vi "Sys config window-Set disabled states.vi"(8 "error in (no error)":errorcluster) -> (0 "error out":errorcluster)   [LabVIEW 2020]
uses:
  Globals/Sys Config window globals.vi
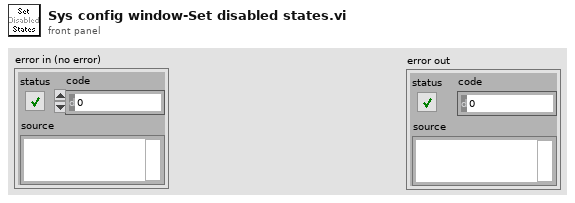
[diagram p1: front panel]
types:
  T1 = enum8{"Enabled", "Disabled", "Disabled and Grayed Out"}
  T2 = typedef "HW config window refs cluster.ctl" = cluster{"VI's reference":refnum<vi>, "menu reference":refnum<k9>, "Pane":refnum<vi>, "Config Tab Control":refnum<vi>, "Triggers sub-tab control":refnum<vi>, "Microscope ID":refnum<vi>, "Microscope Type":refnum<vi>, "Revision Number":refnum<vi>, "Advanced Imaging":refnum<vi>, "Max Allowed Trial Length":refnum<vi>, "Initial Scan Resolution":refnum<vi>, "Initial Acceptance Angle":refnum<vi>, "Initial Laser Wavelength [nm] ":refnum<vi>, "Initial Dwell Time [us]":refnum<vi>, "Error Logging":refnum<vi>, "Performance Monitoring":refnum<vi>, "Ctrl FPGA available":refnum<vi>, "Control HW config":refnum<vi>, "Control System Config":refnum<vi>, "General trigger settings":refnum<vi>, "Trigger HW config":refnum<vi>, "Externalise Triggers":refnum<vi>, "[Triggers output setup]":refnum<vi>, "DAQ FPGA HW Config":refnum<vi>, "DAQ FPGA System Config":refnum<vi>, "Pockels AO":refnum<vi>, "Hard shutter AO":refnum<vi>, "PMT AOs":refnum<vi>, "Galvo AO":refnum<vi>, "Power meter AI":refnum<vi>, "PMT Voltage Lower Limit":refnum<vi>, "PMT Voltage Upper Limit":refnum<vi>, "XYZ Stage Control Config":refnum<vi>, "XY stage available":refnum<vi>, "XY Comms Config Cluster":refnum<vi>, "Y stage available":refnum<vi>, "Y Comms Config Cluster":refnum<vi>, "Z stage available":refnum<vi>, "Z Comms Config Cluster":refnum<vi>, "Encoder available":refnum<vi>, "Encoder":refnum<vi>, "Encoder IP address":refnum<vi>, "Encoder port":refnum<vi>, "Wheel radius (cm)":refnum<vi>, "Demo mode":refnum<vi>, "Swap XY on stage":refnum<vi>, "Number of AODs":refnum<vi>, "Axial MC Supported":refnum<vi>, "MC Supported":refnum<vi>, "Computer MAC add.":refnum<vi>, "Cam VidRec available":refnum<vi>, "Cam VidRec":refnum<vi>, "DO flag-Video record":refnum<vi>, "DO flag-Trial start":refnum<vi>, "AOD Settings (distilled)":refnum<vi>, "Pockels cal.Dwell time (µs)":refnum<vi>, "Pockels cal.Zoom":refnum<vi>, "Current Objective":refnum<vi>, "[Obj. Calib. Settings]":refnum<vi>, "Laser Wavelength":refnum<vi>, "Laser Power Control \nHW config":refnum<vi>, "Laser 1 available":refnum<vi>, "Laser 1 config":refnum<vi>, "Prechirper 1 available":refnum<vi>, "Prechirper 1 config":refnum<vi>, "PreChirp Preset Values":refnum<vi>, "[PreChirper Preset \nCalibration Values]":refnum<vi>, "Prechirper Constants":refnum<vi>}
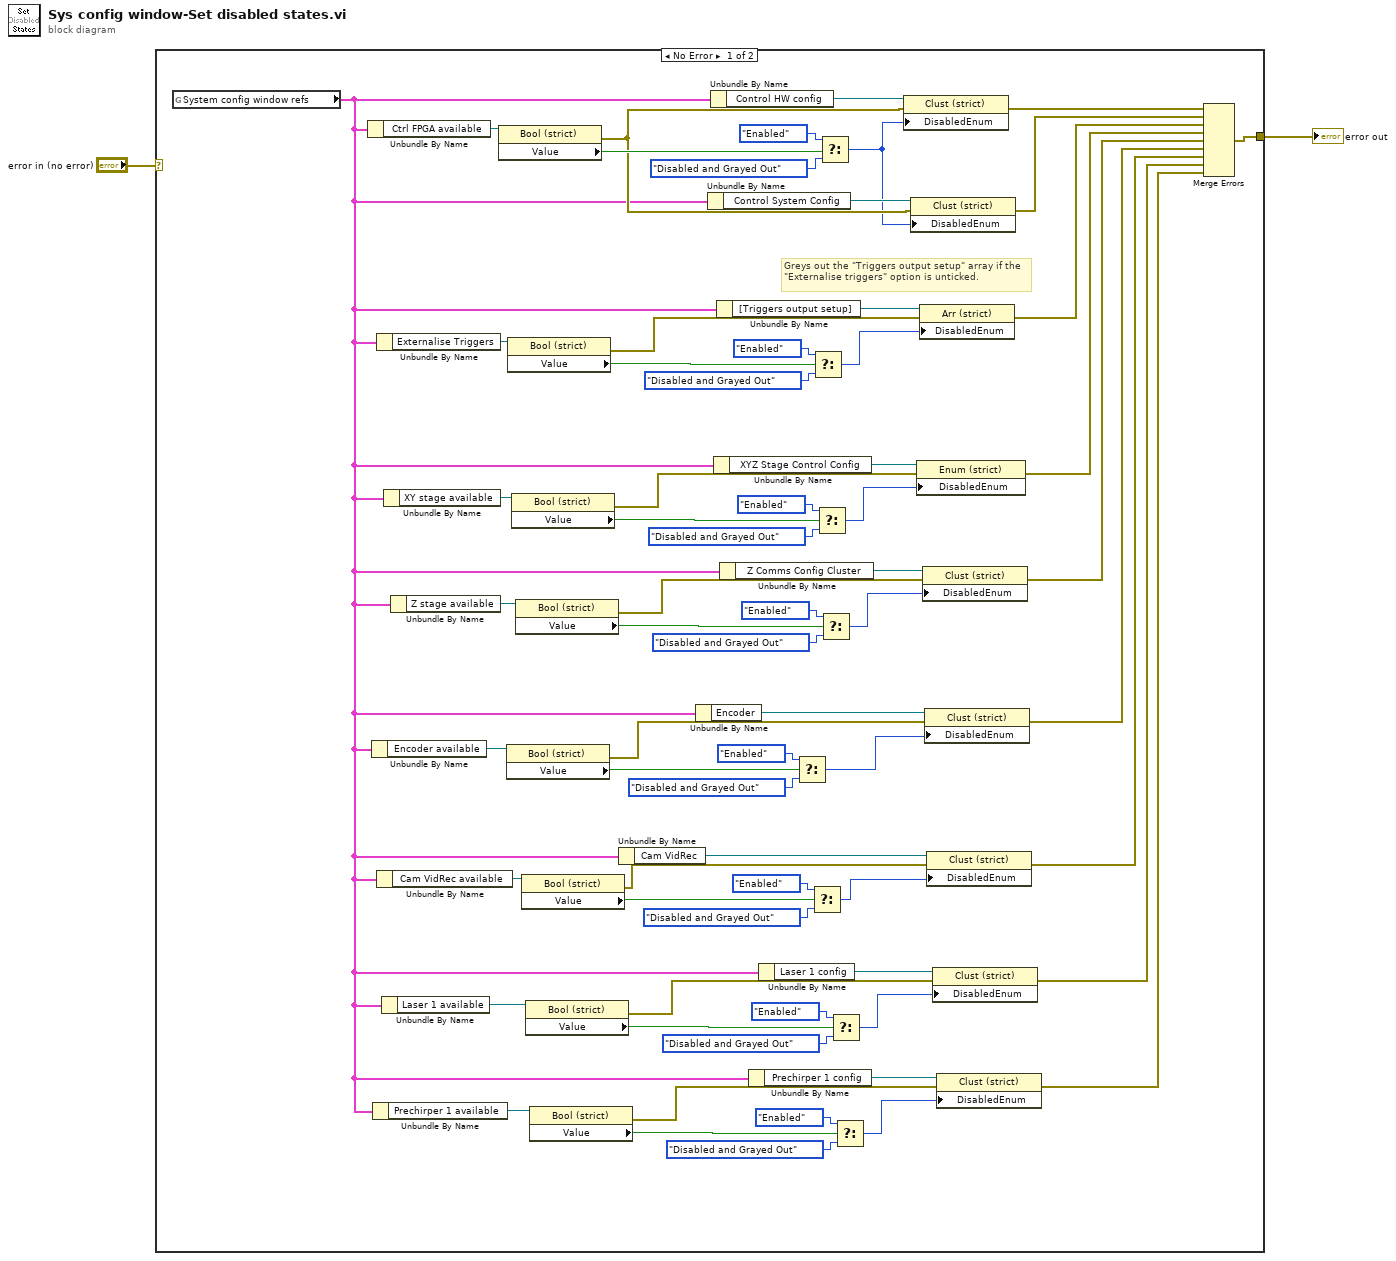
[diagram p0: block diagram]
diagram:
  n1 = case shown="No Error" "error in (no error)" {
    selector: "error in (no error)" -> [_ w71]
    tunnel: [w58 w71] -> w2
    frame No Error {
      # "Greys out the \"Triggers output setup\" array if the \"Externalise triggers\" option is unticked."
      n2 = global read "Sys Config window globals.vi" "System config window refs"() -> (w5:T2)
      n3 = Unbundle By Name(w5) -> ("Ctrl FPGA available"=w47:refnum<vi>)
      n4 = Unbundle By Name(w5) -> ("Encoder available"=w57:refnum<vi>)
      n5 = Unbundle By Name(w5) -> ("Prechirper 1 available"=w23:refnum<vi>)
      n6 = Unbundle By Name(w5) -> ("Externalise Triggers"=w70:refnum<vi>)
      n7 = Unbundle By Name(w5) -> ("Cam VidRec available"=w60:refnum<vi>)
      n8 = Unbundle By Name(w5) -> ("Laser 1 available"=w22:refnum<vi>)
      n9 = Unbundle By Name(w5) -> ("XY stage available"=w39:refnum<vi>)
      n10 = Unbundle By Name(w5) -> ("Z stage available"=w38:refnum<vi>)
      n11 = property class="Bool (strict)"(reference=w47) -> (error out=w6:errorcluster, "Value"=w46:bool)  [unwired: 1 in, 1 out]
      n12 = property class="Bool (strict)"(reference=w57) -> (error out=w51:errorcluster, "Value"=w56:bool)  [unwired: 1 in, 1 out]
      n13 = property class="Bool (strict)"(reference=w70) -> (error out=w64:errorcluster, "Value"=w68:bool)  [unwired: 1 in, 1 out]
      n14 = property class="Bool (strict)"(reference=w39) -> (error out=w45:errorcluster, "Value"=w41:bool)  [unwired: 1 in, 1 out]
      n15 = property class="Bool (strict)"(reference=w38) -> (error out=w32:errorcluster, "Value"=w36:bool)  [unwired: 1 in, 1 out]
      n16 = property class="Bool (strict)"(reference=w60) -> (error out=w53:errorcluster, "Value"=w61:bool)  [unwired: 1 in, 1 out]
      n17 = property class="Bool (strict)"(reference=w22) -> (error out=w16:errorcluster, "Value"=w20:bool)  [unwired: 1 in, 1 out]
      n18 = property class="Bool (strict)"(reference=w23) -> (error out=w29:errorcluster, "Value"=w25:bool)  [unwired: 1 in, 1 out]
      n19 = Unbundle By Name(w5) -> ("Cam VidRec"=w30:refnum<vi>)
      n20 = Unbundle By Name(w5) -> ("Encoder"=w31:refnum<vi>)
      n21 = Unbundle By Name(w5) -> ("Control System Config"=w7:refnum<vi>)
      n22 = Unbundle By Name(w5) -> ("Control HW config"=w50:refnum<vi>)
      n23 = Unbundle By Name(w5) -> ("XYZ Stage Control Config"=w40:refnum<vi>)
      n24 = Unbundle By Name(w5) -> ("[Triggers output setup]"=w69:refnum<vi>)
      n25 = Unbundle By Name(w5) -> ("Z Comms Config Cluster"=w37:refnum<vi>)
      n26 = Unbundle By Name(w5) -> ("Prechirper 1 config"=w24:refnum<vi>)
      n27 = Unbundle By Name(w5) -> ("Laser 1 config"=w21:refnum<vi>)
      n28 = Select(t=T1."Enabled" ("Disabled"), s=w56, f=T1."Disabled and Grayed Out" ("Disabled")) -> (s? t:f=w52:T1)
      n29 = Select(t=T1."Enabled" ("Disabled"), s=w61, f=T1."Disabled and Grayed Out" ("Disabled")) -> (s? t:f=w59:T1)
      n30 = Select(t=T1."Enabled" ("Disabled"), s=w68, f=T1."Disabled and Grayed Out" ("Disabled")) -> (s? t:f=w65:T1)
      n31 = Select(t=T1."Enabled" ("Disabled"), s=w41, f=T1."Disabled and Grayed Out" ("Disabled")) -> (s? t:f=w44:T1)
      n32 = Select(t=T1."Enabled" ("Disabled"), s=w46, f=T1."Disabled and Grayed Out" ("Disabled")) -> (s? t:f=w4:T1)
      n33 = Select(t=T1."Enabled" ("Disabled"), s=w36, f=T1."Disabled and Grayed Out" ("Disabled")) -> (s? t:f=w33:T1)
      n34 = Select(t=T1."Enabled" ("Disabled"), s=w20, f=T1."Disabled and Grayed Out" ("Disabled")) -> (s? t:f=w17:T1)
      n35 = Select(t=T1."Enabled" ("Disabled"), s=w25, f=T1."Disabled and Grayed Out" ("Disabled")) -> (s? t:f=w28:T1)
      n36 = property class="Clust (strict)"(reference=w50, error in=w6, "DisabledEnum"=w4) -> (error out=w15:errorcluster)  [unwired: 1 out]
      n37 = property class="Clust (strict)"(reference=w7, error in=w6, "DisabledEnum"=w4) -> (error out=w3:errorcluster)  [unwired: 1 out]
      n38 = property class="Enum (strict)"(reference=w40, error in=w45, "DisabledEnum"=w44) -> (error out=w14:errorcluster)  [unwired: 1 out]
      n39 = property class="Arr (strict)"(reference=w69, error in=w64, "DisabledEnum"=w65) -> (error out=w8:errorcluster)  [unwired: 1 out]
      n40 = property class="Clust (strict)"(reference=w37, error in=w32, "DisabledEnum"=w33) -> (error out=w13:errorcluster)  [unwired: 1 out]
      n41 = property class="Clust (strict)"(reference=w31, error in=w51, "DisabledEnum"=w52) -> (error out=w12:errorcluster)  [unwired: 1 out]
      n42 = property class="Clust (strict)"(reference=w30, error in=w53, "DisabledEnum"=w59) -> (error out=w11:errorcluster)  [unwired: 1 out]
      n43 = property class="Clust (strict)"(reference=w21, error in=w16, "DisabledEnum"=w17) -> (error out=w10:errorcluster)  [unwired: 1 out]
      n44 = property class="Clust (strict)"(reference=w24, error in=w29, "DisabledEnum"=w28) -> (error out=w9:errorcluster)  [unwired: 1 out]
      n45 = Merge Errors(w15, w3, w8, w14, w13, w12, w11, w10, w9) -> (w58:errorcluster)
    }
    frame Error {
    }
  }
  "error out" <- w2
